vi "ifr2025 Step Through Sequence.vi"(8 "error in (no error)":errorcluster {"code" format="%.0x"}, 9 "Step (Up)":bool=TRUE, 11 "instrument handle":refnum<visa-resource-name>) -> (0 "error out":errorcluster {"code" format="%.0x"}, 2 "Store Num":i16, 3 "instrument handle out":refnum<visa-resource-name>)   [LabVIEW 2009]
doc: "This command allows memory stores to be stepped up or down."
uses:
  Ifr2025_32.dll
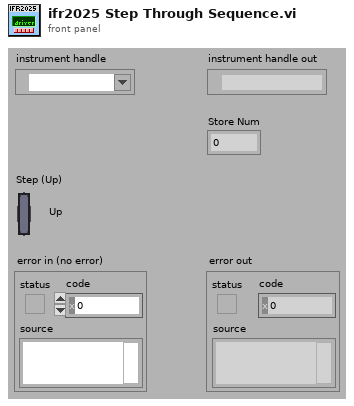
[diagram p1: front panel]
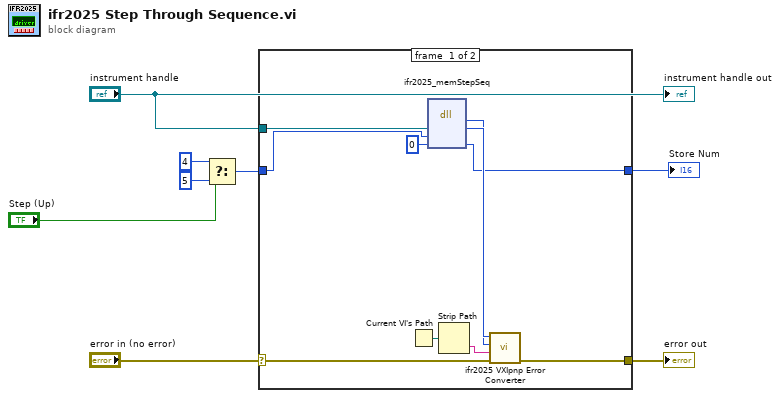
[diagram p0: block diagram]
diagram:
  n1 = Select(t=i16 4, s="Step (Up)", f=i16 5) -> (s? t:f=w2:i16)
  n2 = case shown="No Error" "error in (no error)" {
    selector: "error in (no error)" -> [w13 w19]
    tunnel: [w12 w19] -> w8
    tunnel: "instrument handle" -> [w17 _]
    tunnel: w2 -> [w11 _]
    tunnel: [w9 _] -> w1
    frame #0 {
      n3 = Current VI's Path() -> (path=w18:path)
      n4 = dll-call lib="P:/inst/Marconi 2024 Signal Generator/source/labview/ifr2025/ifr2025/ifr2025_*.*" fn="ifr2025_memStepSeq"("vi"=w17, "Step"=w11, "Store Num"=i16 0) -> (w15:i32, "vi"=w16:u32, "Store Num"=w9:i16)  [unwired: 4 in, 2 out]
      n5 = Strip Path(path=w18) -> (name=w14:string)  [unwired: 1 out]
      n6 = call "ifr2025 VXIpnp Error Converter.vi"("error in (no error)"=w13, "name of VI (\"\")"=w14, "CVI error code (0)"=w15, "instrument handle"=w16) -> ("error out"=w12:errorcluster)  [unwired: 7 out]
    }
    frame #1 {
    }
  }
  "error out" <- w8
  "Store Num" <- w1
  "instrument handle out" <- "instrument handle"
